vi "U8.vi"(1 "Numeric Input":u8) -> (0 "Numeric Output":u8)   [LabVIEW 2012]
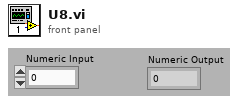
[diagram p1: front panel]
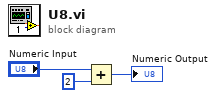
[diagram p0: block diagram]
diagram:
  n1 = Add(x="Numeric Input", y=u8 2) -> (x+y=→"Numeric Output":u8)
